vi "get_error_codes.vi"(8 "Error in 2":errorcluster caption="Error in (no error)") -> (0 "Error out 2":errorcluster, 3 "Error Codes":string)   [LabVIEW 2018]
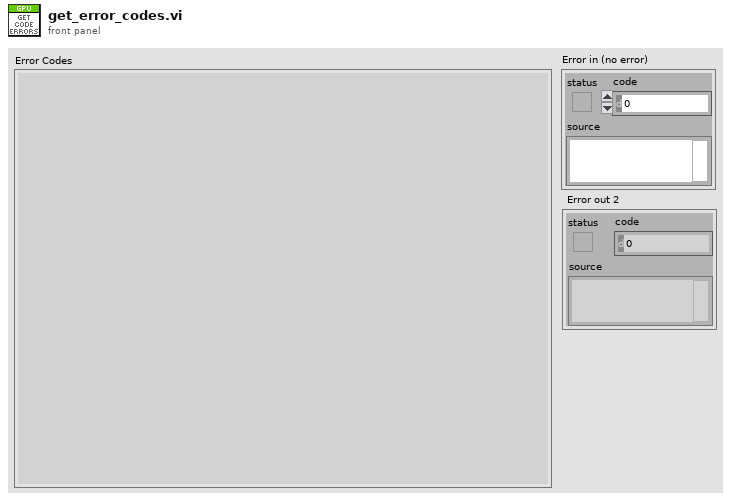
[diagram p1: front panel]
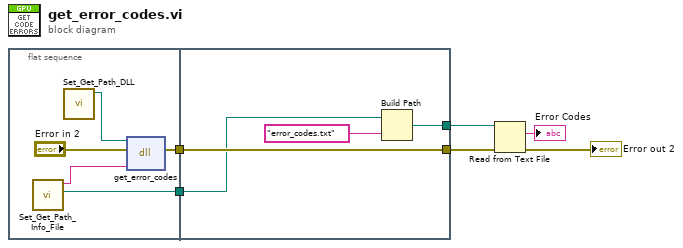
[diagram p0: block diagram]
diagram:
  n1 = flat-sequence {
    tunnel: [w10] -> w3
    tunnel: [w7] -> w1
    tunnel: [w15] -> w5
    tunnel: w3 -> [w15]
    tunnel: [w13] -> w2
    tunnel: w1 -> [w12]
    frame #0 {
      n2 = call "Set_Get_Path_Info_File.vi"() -> ("Info File Path Out"=w7:path, "Info Path File Out"=w8:string)  [unwired: 10 in]
      n3 = call "Set_Get_Path_DLL.vi"() -> ("path DLL Out"=w9:path)  [unwired: 11 in]
      n4 = dll-call lib="C:/Users/AUTIS/Documents/TFG/Proyecto/LabVIEW_PRUEBAS/VIs/Utilidades/DLL/SR_GPU_TOOLKIT.dll" fn="get_error_codes"(path in=w9, error in="Error in 2", "url"=w8) -> (error out=w10:errorcluster)  [unwired: 3 in, 1 out]
    }
    frame #1 {
      n5 = Build Path(base path=w12, name or relative path="error_codes.txt") -> (appended path=w13:path)
    }
  }
  n6 = Read from Text File(file (use dialog)=w2, error in=w5) -> (text=→"Error Codes":string, error out=→"Error out 2":errorcluster)  [unwired: 2 in, 2 out]
